vi "SA40144D.20210528 Devices + BG.vi"() -> ()   [LabVIEW 2020]
uses:
  <vilib>/Analysis/baseanly.llb/Mean (DBL).vi
  <userlib>/_OpenG.lib/file/file.llb/Build Path - Traditional__ogtk.vi
  <userlib>/LevyLab/LV to ITX/Data/Data.lvclass
  <userlib>/LevyLab/XY Utilities/xy_utilities.lvlib
  <vilib>/Analysis/NI_AALBase.lvlib
panel:
  out "G2T BG vs t":T1(graph)
  in  "Temps to keep (Lifespan)":i32=26
  out "Lifespan vs Temp (hrs)":cluster{i32[], dbl[]}[](graph)
  out "E_a":dbl[](array[numeric])
  out "Arrhenius":T1(graph)
  in  "Temps to keep (Arrhenius fit)":i32=26
  out "G2T vs t":T1(graph)
  out "G4T vs t":T1(graph)
  out "G2T vs t 2D":T1(graph)
  out "G4T vs t  2D":T1(graph)
  out "Temp vs t":T1(graph)
  in  "Source Voltage":dbl=0.1
  in  "Init Temp":i32=275
  in  "Temp Step":i32=5
  in  "Final Temp":i32=400
  in  "Data File":path=path "G:/My Drive/ansom/Data/PPMS 2/SA40144D.20210601/00 - Air Test/SA40144D.20210601.275K.dat"
  in  "Trimming":i32=400
  in  "Update":bool
  in  "OK":bool
  out "error out":errorcluster
  in  "error in (no error)":errorcluster
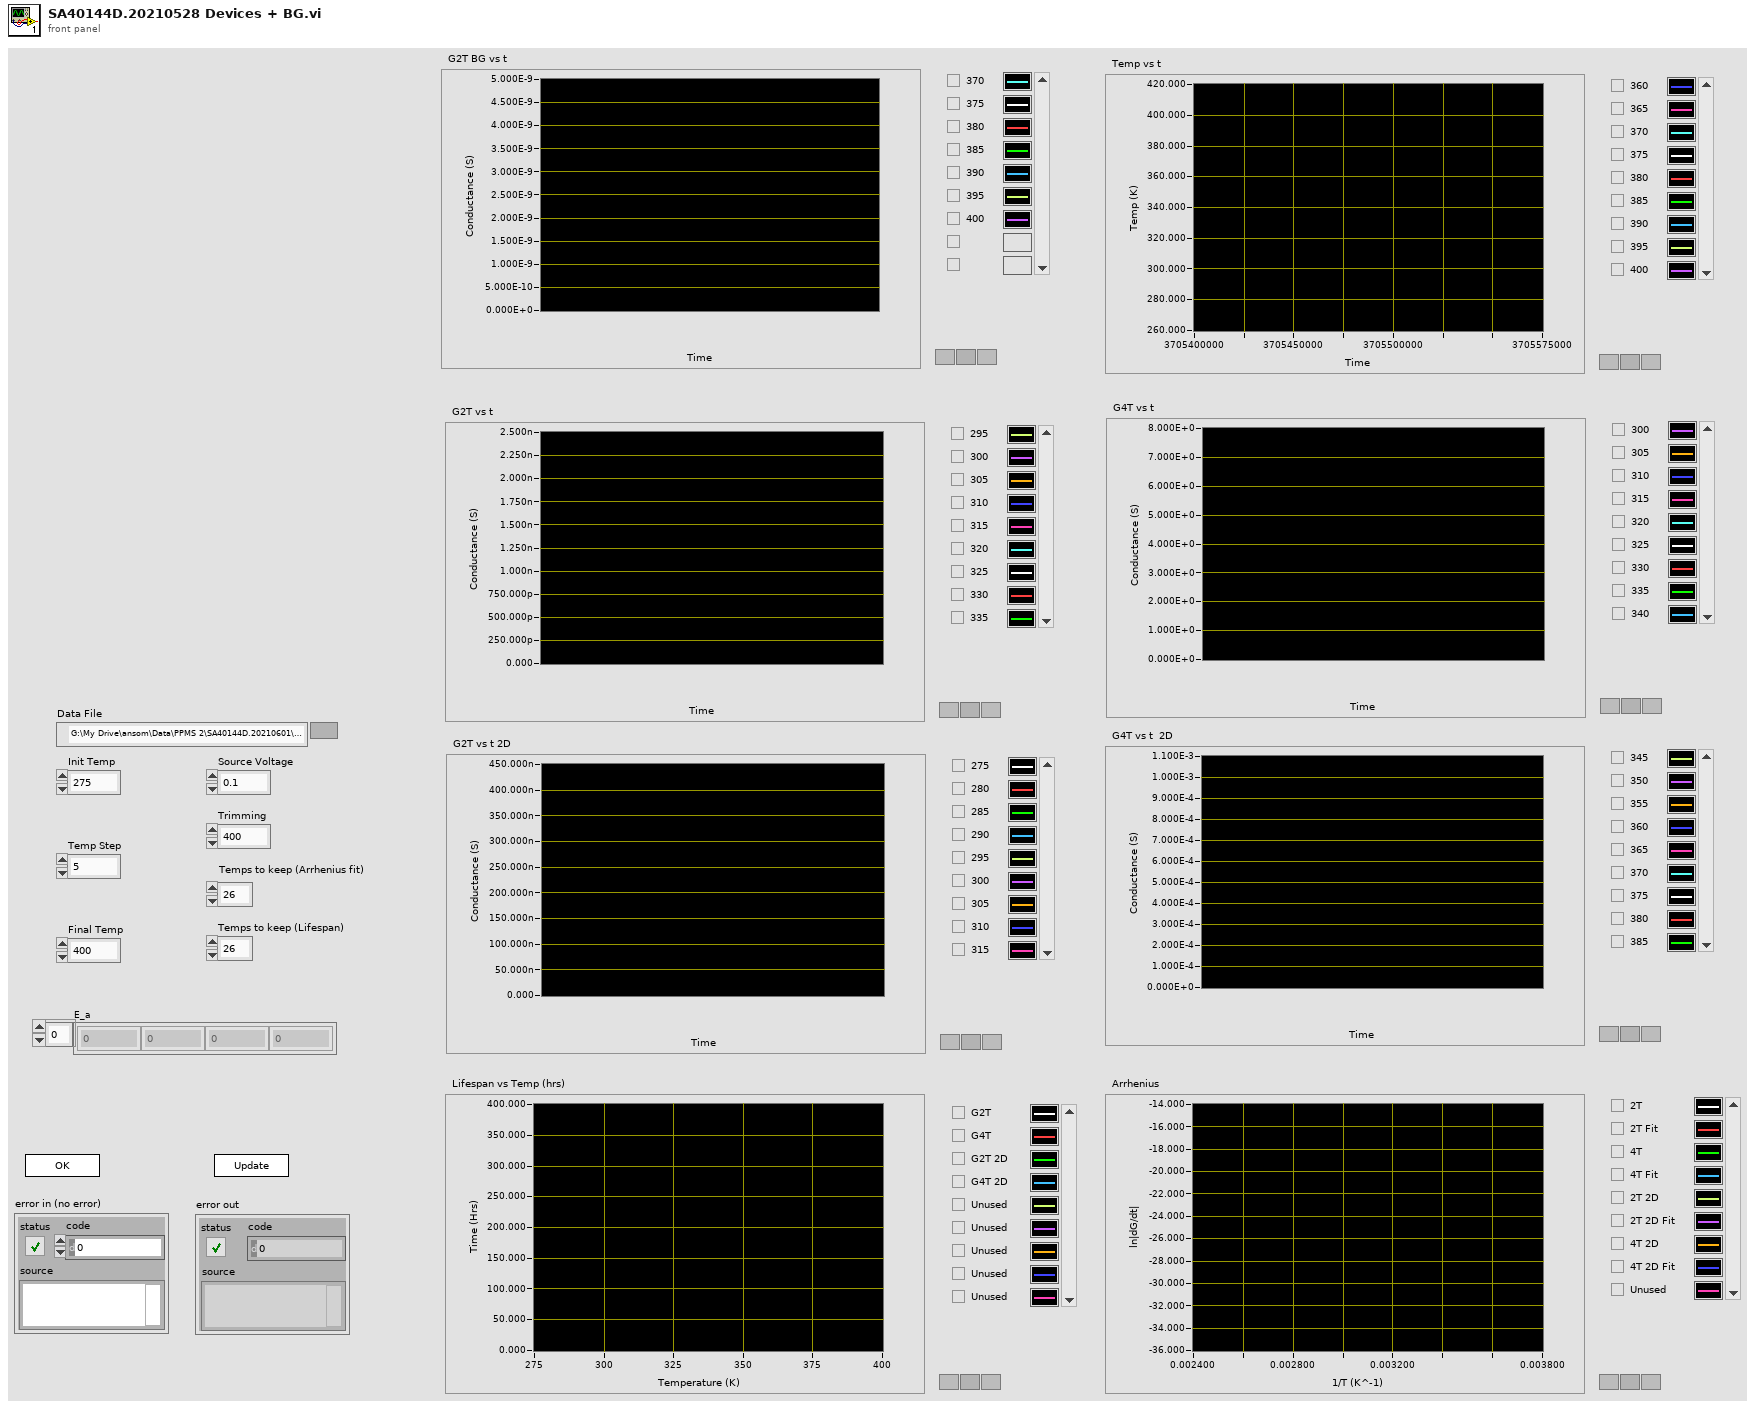
[diagram p1: front panel]
types:
  T1 = cluster{"Data":dbl[], "Best Exponential Fit":dbl[]}[]
  T2 = enum32{"Invalid", "Standard", "Closed", "Hidden", "Minimized", "Maximized"}
  T3 = enum32{"invalid app kind", "Development System", "Run Time System", "Student Edition", "Embedded LabVIEW", "Evaluation", "Custom"}
  T4 = cluster{"Core":cluster{"Current VI Reference":refnum<vi>, "Close Panel on Exit?":bool}, "G2T 1D":cluster{dbl[], dbl[]}[], "G4T 1D":cluster{dbl[], dbl[]}[], "G2T 2D":cluster{dbl[], dbl[]}[], "G4T 2D":cluster{dbl[], dbl[]}[], "Temp":cluster{dbl[], dbl[]}[], "G2T BG":cluster{dbl[], dbl[]}[], "Source Voltage":dbl, "Final Temp":i32, "Init Temp":i32, "Temp Step":i32, "Data File":path, "Trimming":i32}
  T5 = cluster{"Current VI Reference":refnum<vi>, "Close Panel on Exit?":bool}
  T6 = typedef "Data.lvclass/Dictionary--cluster.ctl" = cluster{"key":string, "value":variant}
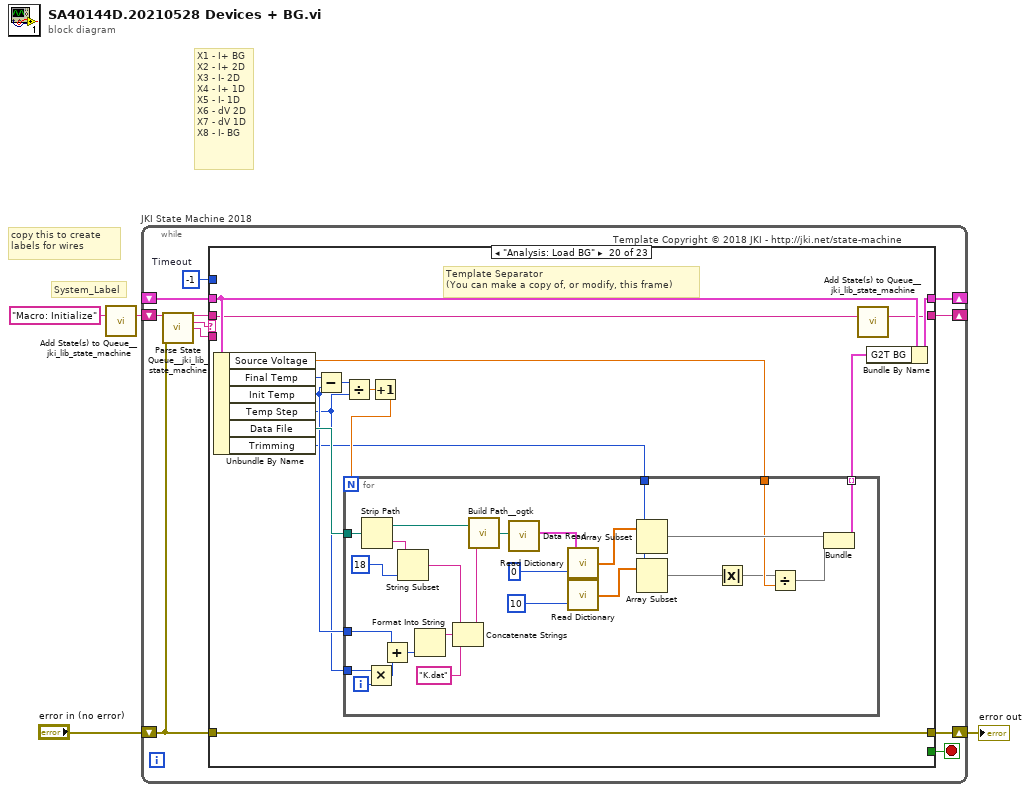
[diagram p0: block diagram]
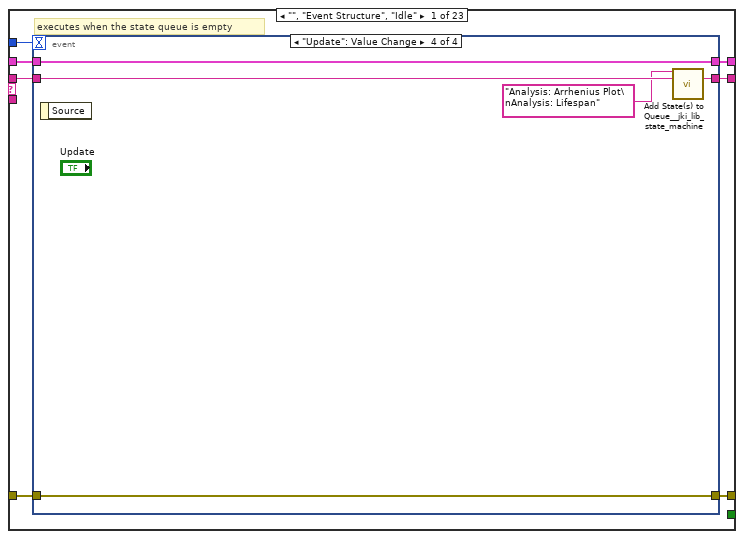
[diagram p2: hidden frame]
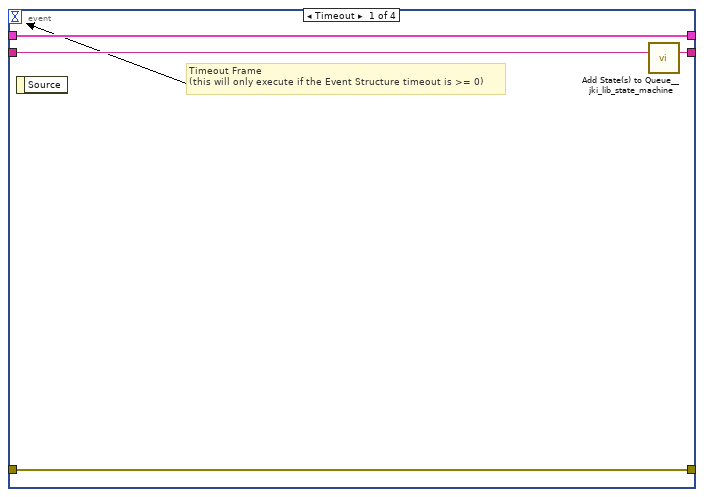
[diagram p3: hidden frame]
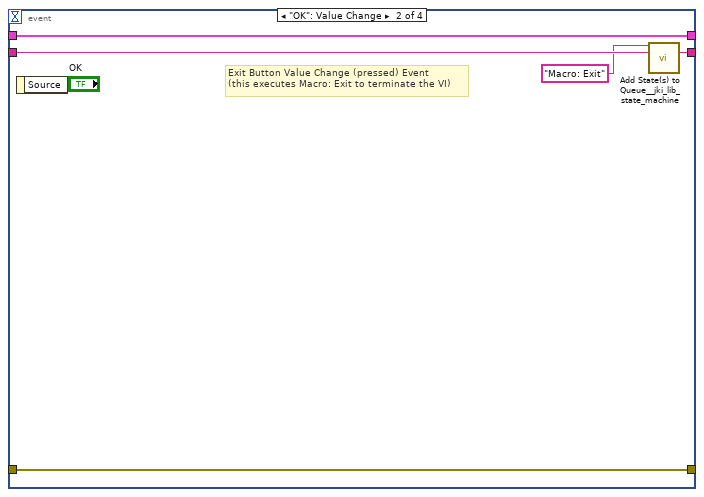
[diagram p4: hidden frame]
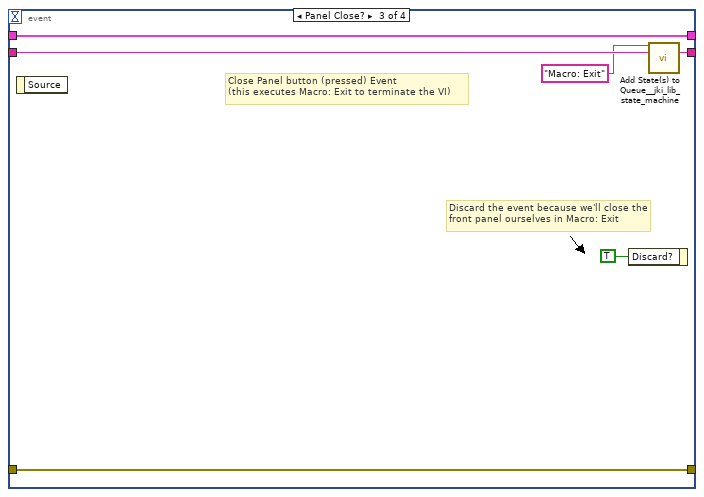
[diagram p5: hidden frame]
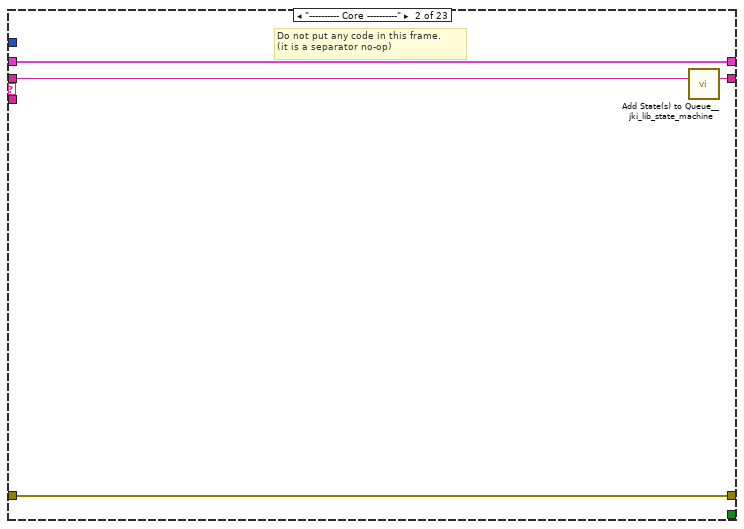
[diagram p6: hidden frame]
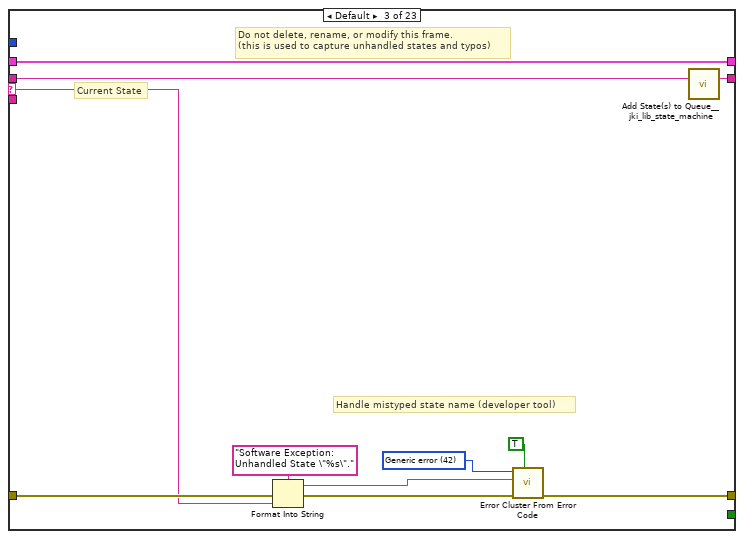
[diagram p7: hidden frame]
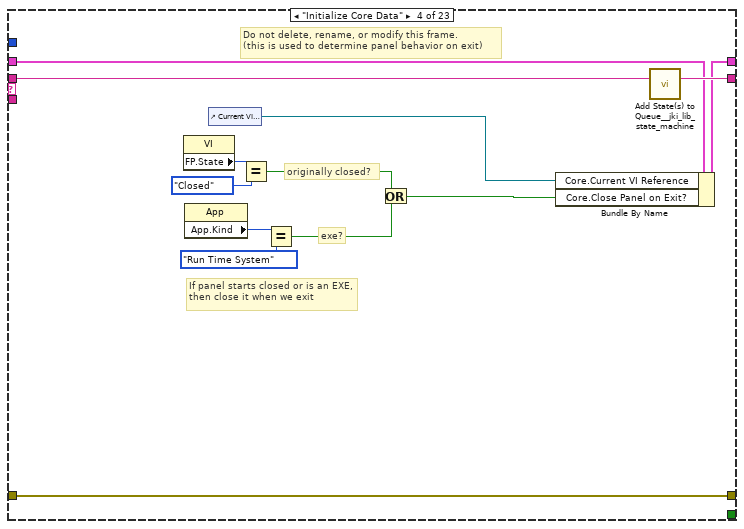
[diagram p8: hidden frame]
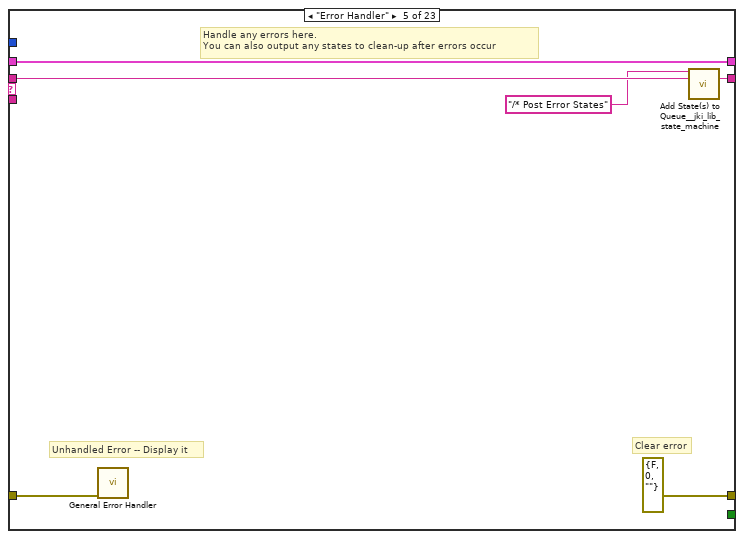
[diagram p9: hidden frame]
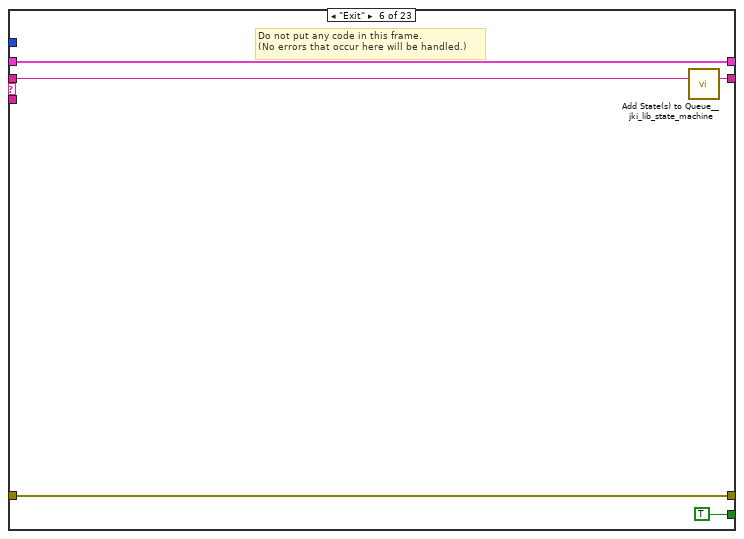
[diagram p10: hidden frame]
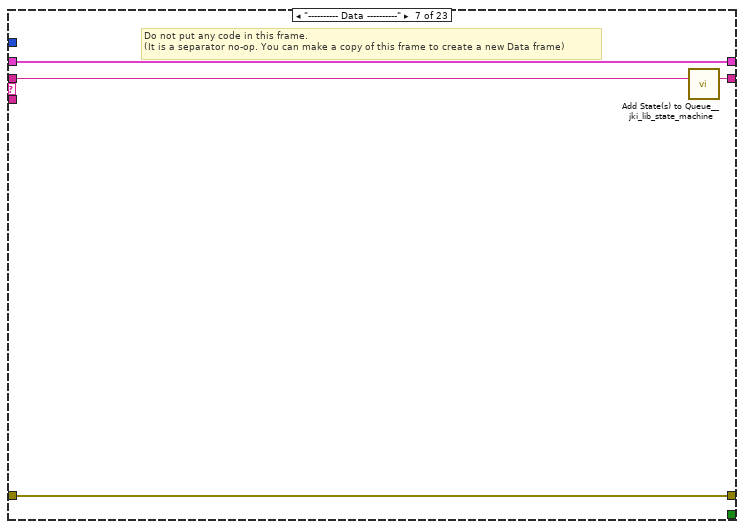
[diagram p11: hidden frame]
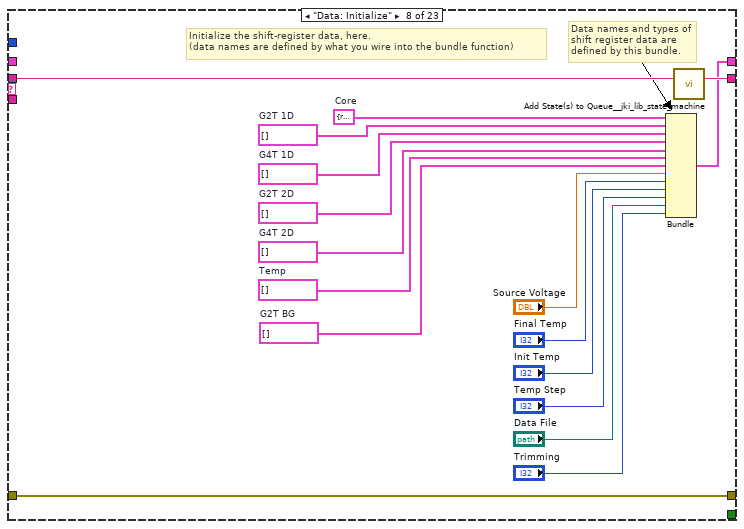
[diagram p12: hidden frame]
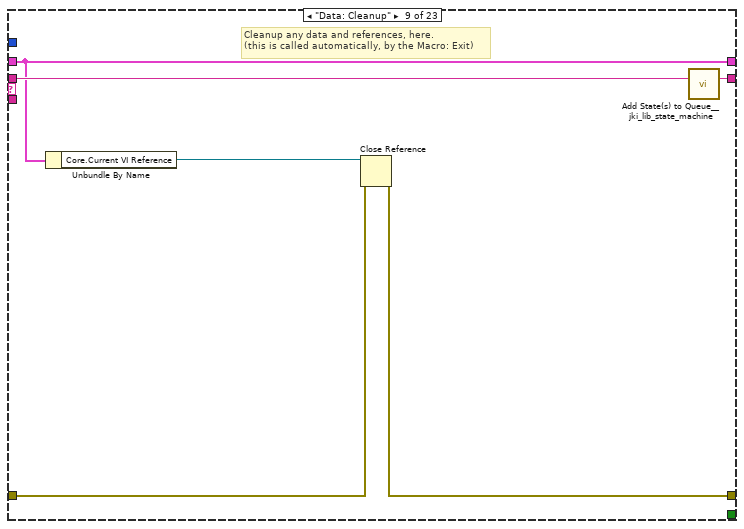
[diagram p13: hidden frame]
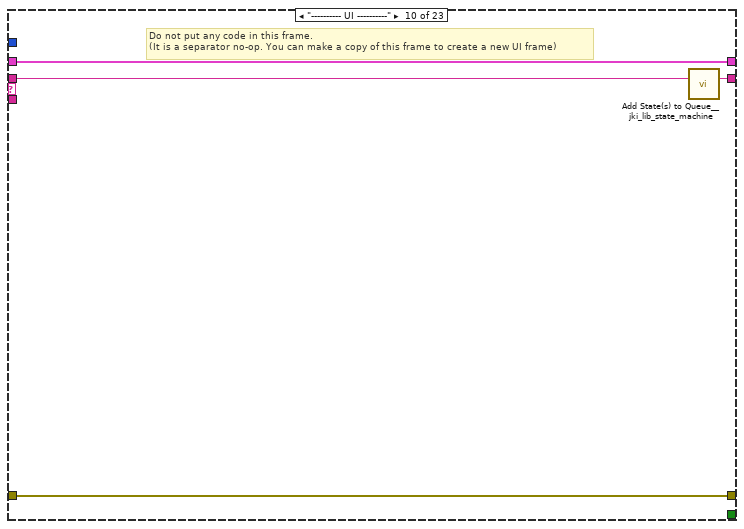
[diagram p14: hidden frame]
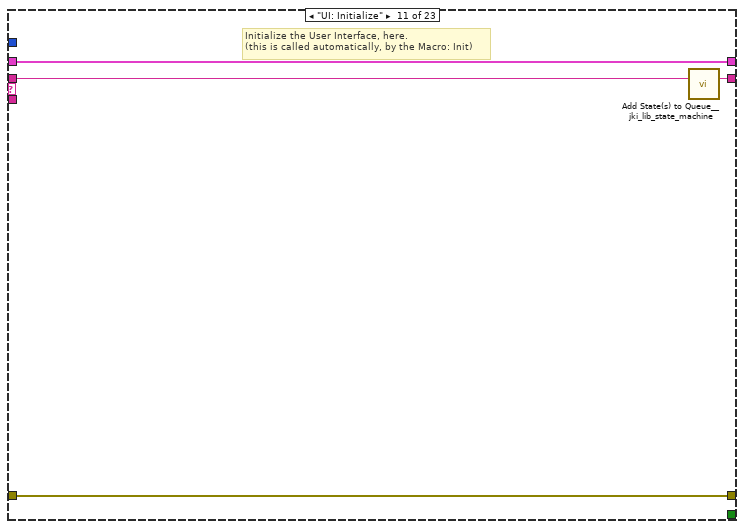
[diagram p15: hidden frame]
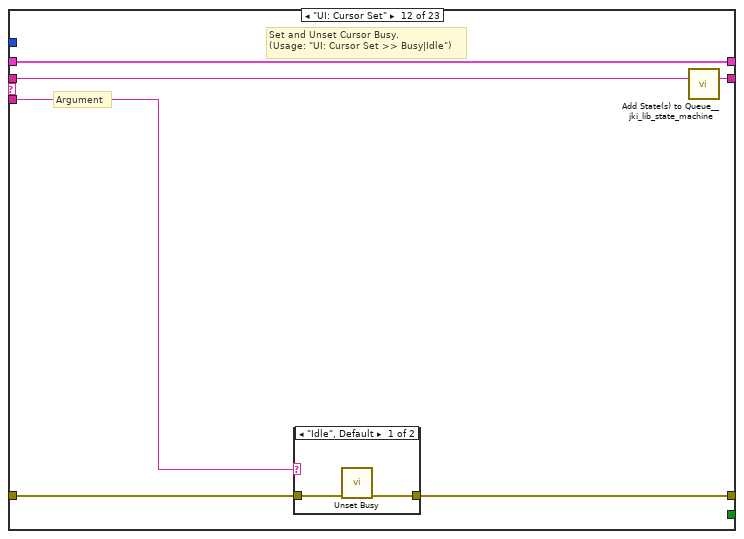
[diagram p16: hidden frame]
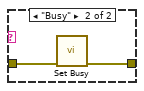
[diagram p17: hidden frame]
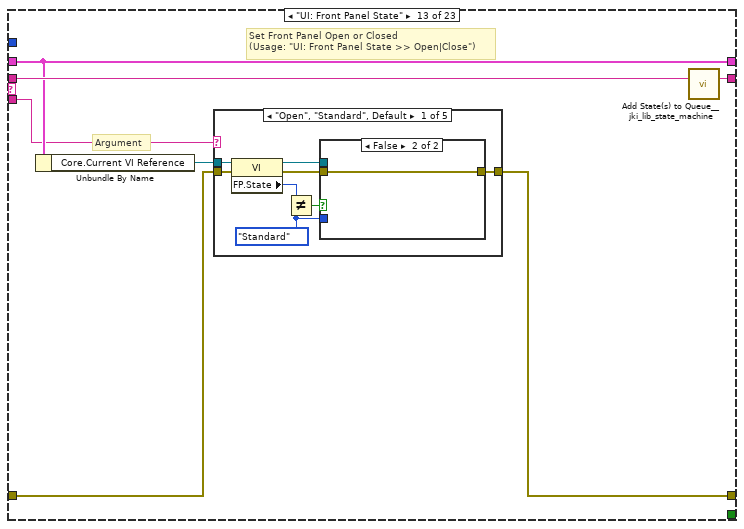
[diagram p18: hidden frame]
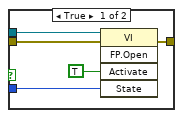
[diagram p19: hidden frame]
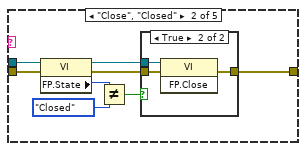
[diagram p20: hidden frame]
diagram:
  # "X1 - I+ BG\nX2 - I+ 2D\nX3 - I- 2D\nX4 - I+ 1D\nX5 - I- 1D\nX6 - dV 2D\nX7 - dV 1D\nX8 - I- BG"
  # "copy this to create labels for wires"
  # "System_Label"
  n1 = call <vilib>:"Add State(s) to Queue__jki_lib_state_machine.vi"("State(s) in (\"\")"="Macro: Initialize") -> ("States Out"=w4:string)  [unwired: 14 in]
  n2 = while "JKI State Machine 2018" {
    shift-right: [w8] -> _
    shift-left: _ -> [w7]
    shift-right: [w11] -> w1
    shift-left: "error in (no error)" -> [w5]
    shift-right: [w10] -> _
    shift-left: w4 -> [w12]
    stop <- w9 stop-if-true
    w6 = -1  # Timeout
    # "Template Copyright © 2018 JKI - http://jki.net/state-machine"
    n3 = call <vilib>:"Parse State Queue__jki_lib_state_machine.vi"("State Queue"=w12, "Error In (no error)"=w5) -> ("Remaining States"=w14:string, "Current State"=w15:string, "Arguments"=w13:string)  [unwired: 11 in]
    n4 = case shown="\"Analysis: Load BG\"" w15 {
      selector: w15 -> [_ _ w47 _ _ _ _ _ _ _ _ _ _ _ _ _ _ _ _ _ _ _ _]
      tunnel: w14 -> [w22 w46 w51 w70 w76 w81 w85 w102 w108 w112 w116 w122 w133 w202 w207 w217 w221 w238 w290 w323 w373 w417 w474]
      tunnel: w13 -> [_ _ _ _ _ _ _ _ _ _ _ w117 w127 _ _ _ _ _ _ _ _ _ _]
      tunnel: w7 -> [w20 w43 w49 w63 w73 w79 w82 _ w103 w109 w114 w120 w129 w199 w204 w214 w218 w232 w275 w325 w370 w414 w454]
      tunnel: [w19 w44 w53 w67 errorcluster {"status"=FALSE, "code"=0, "source"=""} ("error out") w78 w83 w99 w104 w110 w113 w118 w130 w200 w205 w215 w219 w234 w288 w337 w371 w415 w472] -> w11
      tunnel: w5 -> [w18 w44 w52 w67 w72 w78 w83 w99 w105 w110 w113 w119 w131 w200 w205 w215 w219 w234 w288 w337 w371 w415 w472]
      tunnel: [w21 w45 w50 w69 w75 w80 w84 w101 w107 w111 w115 w121 w132 w201 w206 w216 w220 w237 w289 w324 w372 w416 w473] -> w10
      tunnel: [_ _ _ _ _ TRUE _ _ _ _ _ _ _ _ _ _ _ _ _ _ _ _ _] -> w9
      tunnel: [w17 w43 w49 w68 w73 w79 w82 w100 w103 w109 w114 w120 w129 w199 w204 w214 w218 w233 w276 w326 w370 w414 w454] -> w8
      tunnel: w6 -> [w16 _ _ _ _ _ _ _ _ _ _ _ _ _ _ _ _ _ _ _ _ _ _]
      frame "", "Event Structure", "Idle" {
        # "executes when the state queue is empty"
        n5 = event shown="[3] \"Update\": Value Change" {
          selector: _ -> [_ _ _ _]
          dyn-events: _ -> [_ _ _ _]
          timeout: w16 -> [_ _ _ _]
          tunnel: w22 -> [w26 w31 w37 w41]
          tunnel: [w25 w30 w36 w40] -> w21
          tunnel: w20 -> [w23 w28 w34 w42]
          tunnel: [w24 w29 w35 w38] -> w19
          tunnel: w18 -> [w24 w29 w35 w38]
          tunnel: [w23 w28 w34 w42] -> w17
          event Timeout {
            # "Timeout Frame\n(this will only execute if the Event Structure timeout is >= 0)"
            n6 = event-data() -> ()  [unwired: 1 in, 1 out]
            n7 = call <vilib>:"Add State(s) to Queue__jki_lib_state_machine.vi"("State(s) in (\"\")"=w26) -> ("States Out"=w25:string)  [unwired: 14 in]
          }
          event "OK": Value Change {
            # "Exit Button Value Change (pressed) Event\n(this executes Macro: Exit to terminate the VI)"
            n8 = event-data() -> ()  [unwired: 1 in, 1 out]
            n9 = call <vilib>:"Add State(s) to Queue__jki_lib_state_machine.vi"("State(s) in Front (\"\")"="Macro: Exit", "State(s) in (\"\")"=w31) -> ("States Out"=w30:string)  [unwired: 13 in]
          }
          event Panel Close? {
            # "Discard the event because we'll close the front panel ourselves in Macro: Exit"
            # "Close Panel button (pressed) Event\n(this executes Macro: Exit to terminate the VI)"
            n10 = event-data() -> ()  [unwired: 1 in, 1 out]
            n11 = event-data("Discard?"=TRUE) -> ()  [unwired: 1 in, 1 out]
            n12 = call <vilib>:"Add State(s) to Queue__jki_lib_state_machine.vi"("State(s) in Front (\"\")"="Macro: Exit", "State(s) in (\"\")"=w37) -> ("States Out"=w36:string)  [unwired: 13 in]
          }
          event "Update": Value Change {
            n13 = event-data() -> ()  [unwired: 1 in, 1 out]
            n14 = call <vilib>:"Add State(s) to Queue__jki_lib_state_machine.vi"("State(s) in Front (\"\")"="Analysis: Arrhenius Plot\nAnalysis: Lifespan" ("State(s) in Front (\"\")"), "State(s) in (\"\")"=w41) -> ("States Out"=w40:string)  [unwired: 13 in]
          }
        }
      }
      frame "---------- Core ----------" {
        # "Do not put any code in this frame.\n(it is a separator no-op)"
        n15 = call <vilib>:"Add State(s) to Queue__jki_lib_state_machine.vi"("State(s) in (\"\")"=w46) -> ("States Out"=w45:string)  [unwired: 14 in]
      }
      frame Default {
        w56 = 42 items=["No error", "Argument error", "Memory is full", "Out of zone", "End of file", "File already open", "Generic file I/O error", "File not found", "File permission error", "Disk is full", "Duplicate path", "Too many files open", "System feature not enabled", "Resource file not found", "Cannot add resource", "Resource not found", "Image not found", "Image memory error", "Pen does not exist", "Config type invalid", "Config token not found", "Config parse error", "Config memory error", "Bad external code format", "Bad external code offset", "External code not present", "Null window", "Destroy window error", "Null menu", "Print aborted", "Bad print record", "Print driver error", "Windows error during printing", "Memory error during printing", "Print dialog error", "Generic print error", "Invalid device refnum", "Device not found", "Device parameter error", "Device unit error", "Cannot open device", "Device call aborted", "Generic error", "Cancelled by user", "Object ID too low", "Object ID too high", "Object not in heap", "Unknown heap", "Unknown object (invalid DefProc)", "Unknown object (DefProc not in table)", "Message out of range", "Invalid (null) method", "Unknown message", "Manager call not supported", "Bad address", "Network operation in progress", "Network operation timed out", "Connection is busy", "Network attribute not supported", "Network error", "Address in use", "System out of memory", "Connection aborted", "Connection refused", "Not connected", "Already connected", "Connection closed", "Initialization error (interapplication manager)", "Bad occurrence", "Wait on unbound occurrence handler", "Occurrence queue overflow", "Datalog type conflict", "Unused", "Unrecognized type (interapplication manager)", "Memory corrupt", "Failed to make temporary DLL", "Old CIN version", "Drag socket not found", "Failed to load drop-object", "Failed to register OLE object", "Failed to release OLE object", "Format specifier type mismatch", "Unknown format specifier", "Too few format specifiers", "Too many format specifiers", "Scan failed", "Newer CIN version", "Error converting to variant", "Runtime menu error", "Password tampered", "Variant attribute not found", "Incompatible variant data type", "Event data is not available", "Event Store is not present", "Occurrence is not found", "Event Queue is not created", "Event info is not available", "Refnum passed is NULL", "Error retrieving Class GUID", "Error retrieving CoClass GUID", "Error retrieving TypeLib GUID.", "Bad built application magic bytes.", "Specific driver is different from the specific driver associated with the Logical Name.", "There is no session opened to the class driver.", "Max Error", "MAX - Error with config objects", "MAX - Error loading configuration", "MAX - Group not supported"]
        # "Current State"
        # "Do not delete, rename, or modify this frame.\n(this is used to capture unhandled states and typos)"
        # "Handle mistyped state name (developer tool)"
        n16 = Format Into String(format string="Software Exception: Unhandled State \"%s\"." ("message"), error in=w52, w47) -> (resulting string=w55:string, error out=w54:errorcluster)  [unwired: 1 in]
        n17 = call <vilib>:"Error Cluster From Error Code.vi"("show call chain? (False)"=TRUE, "error in (no error)"=w54, "error message (\"\")"=w55, "error code (0)"=w56) -> ("error out"=w53:errorcluster)  [unwired: 5 in]
        n18 = call <vilib>:"Add State(s) to Queue__jki_lib_state_machine.vi"("State(s) in (\"\")"=w51) -> ("States Out"=w50:string)  [unwired: 14 in]
      }
      frame "Initialize Core Data" {
        # "Do not delete, rename, or modify this frame.\n(this is used to determine panel behavior on exit)"
        # "originally closed?"
        # "exe?"
        # "If panel starts closed or is an EXE, then close it when we exit"
        n19 = property class="VI"() -> ("FP.State"=w60:T2)  [unwired: 2 in, 2 out]
        n20 = property class="App"() -> ("App.Kind"=w66:T3)  [unwired: 2 in, 2 out]
        n21 = control-ref of="Current VI Reference"() -> (w61:refnum<vi>)
        n22 = Equal?(x=w60, y=T2."Closed" ("Front Panel Window:State")) -> (x = y?=w58:bool)
        n23 = Equal?(x=w66, y=T3."Run Time System" ("Application:Kind")) -> (x = y?=w64:bool)
        n24 = Or(x=w58, y=w64) -> (x .or. y?=w62:bool)
        n25 = Bundle By Name(cluster=w63, "Core.Current VI Reference"=w61, "Core.Close Panel on Exit?"=w62) -> (w68:T4)
        n26 = call <vilib>:"Add State(s) to Queue__jki_lib_state_machine.vi"("State(s) in (\"\")"=w70) -> ("States Out"=w69:string)  [unwired: 14 in]
      }
      frame "Error Handler" {
        # "Unhandled Error -- Display it"
        # "Handle any errors here.\nYou can also output any states to clean-up after errors occur"
        # "Clear error"
        n27 = call <vilib>:"General Error Handler.vi"("error in (no error)"=w72) -> ()  [unwired: 10 in, 5 out]
        n28 = call <vilib>:"Add State(s) to Queue__jki_lib_state_machine.vi"("State(s) in Front (\"\")"="/* Post Error States", "State(s) in (\"\")"=w76) -> ("States Out"=w75:string)  [unwired: 13 in]
      }
      frame "Exit" {
        # "Do not put any code in this frame.\n(No errors that occur here will be handled.)"
        n29 = call <vilib>:"Add State(s) to Queue__jki_lib_state_machine.vi"("State(s) in (\"\")"=w81) -> ("States Out"=w80:string)  [unwired: 14 in]
      }
      frame "---------- Data ----------" {
        # "Do not put any code in this frame.\n(It is a separator no-op. You can make a copy of this frame to create a new Data frame)"
        n30 = call <vilib>:"Add State(s) to Queue__jki_lib_state_machine.vi"("State(s) in (\"\")"=w85) -> ("States Out"=w84:string)  [unwired: 14 in]
      }
      frame "Data: Initialize" {
        w86 = cluster{dbl[], dbl[]}[] []  # G2T BG
        w87 = cluster{dbl[], dbl[]}[] []  # Temp
        w96 = cluster{dbl[], dbl[]}[] []  # G4T 2D
        w95 = cluster{dbl[], dbl[]}[] []  # G2T 2D
        w94 = cluster{dbl[], dbl[]}[] []  # G4T 1D
        w93 = cluster{dbl[], dbl[]}[] []  # G2T 1D
        w98 = T5 {"Current VI Reference"=refnum, "Close Panel on Exit?"=FALSE}  # Core
        # "Data names and types of shift register data are defined by this bundle."
        # "Initialize the shift-register data, here.\n(data names are defined by what you wire into the bundle function)"
        n31 = Bundle("Core"=w98, "G2T 1D"=w93, "G4T 1D"=w94, "G2T 2D"=w95, "G4T 2D"=w96, "Temp"=w87, "G2T BG"=w86, "Source Voltage"="Source Voltage", "Final Temp"="Final Temp", "Init Temp"="Init Temp", "Temp Step"="Temp Step", "Data File"="Data File", "Trimming"="Trimming") -> (w100:T4)  [unwired: 1 in]
        n32 = call <vilib>:"Add State(s) to Queue__jki_lib_state_machine.vi"("State(s) in (\"\")"=w102) -> ("States Out"=w101:string)  [unwired: 14 in]
      }
      frame "Data: Cleanup" {
        # "Cleanup any data and references, here.\n(this is called automatically, by the Macro: Exit)"
        n33 = Unbundle By Name(w103) -> ("Core.Current VI Reference"=w106:refnum<vi>)
        n34 = Close Reference(reference=w106, error in (no error)=w105) -> (error out=w104:errorcluster)
        n35 = call <vilib>:"Add State(s) to Queue__jki_lib_state_machine.vi"("State(s) in (\"\")"=w108) -> ("States Out"=w107:string)  [unwired: 14 in]
      }
      frame "---------- UI ----------" {
        # "Do not put any code in this frame.\n(It is a separator no-op. You can make a copy of this frame to create a new UI frame)"
        n36 = call <vilib>:"Add State(s) to Queue__jki_lib_state_machine.vi"("State(s) in (\"\")"=w112) -> ("States Out"=w111:string)  [unwired: 14 in]
      }
      frame "UI: Initialize" {
        # "Initialize the User Interface, here.\n(this is called automatically, by the Macro: Init)"
        n37 = call <vilib>:"Add State(s) to Queue__jki_lib_state_machine.vi"("State(s) in (\"\")"=w116) -> ("States Out"=w115:string)  [unwired: 14 in]
      }
      frame "UI: Cursor Set" {
        # "Argument"
        # "Set and Unset Cursor Busy.\n(Usage: \"UI: Cursor Set >> Busy|Idle\")"
        n38 = case shown="\"Idle\", Default" w117 {
          tunnel: w119 -> [w124 w126]
          tunnel: [w123 w125] -> w118
          frame "Idle", Default {
            n39 = call <vilib>:"Unset Busy.vi"("error in (no error)"=w124) -> ("error out"=w123:errorcluster)  [unwired: 10 in]
          }
          frame "Busy" {
            n40 = call <vilib>:"Set Busy.vi"("error in (no error)"=w126) -> ("error out"=w125:errorcluster)  [unwired: 9 in, 1 out]
          }
        }
        n41 = call <vilib>:"Add State(s) to Queue__jki_lib_state_machine.vi"("State(s) in (\"\")"=w122) -> ("States Out"=w121:string)  [unwired: 14 in]
      }
      frame "UI: Front Panel State" {
        # "Argument"
        # "Set Front Panel Open or Closed\n(Usage: \"UI: Front Panel State >> Open|Close\")"
        n42 = Unbundle By Name(w129) -> ("Core.Current VI Reference"=w128:refnum<vi>)
        n43 = case shown="\"Open\", \"Standard\", Default" w127 {
          tunnel: w131 -> [w139 w154 w165 w178 w191]
          tunnel: [w141 w155 w167 w180 w193] -> w130
          tunnel: w128 -> [w140 w152 w166 w179 w192]
          frame "Open", "Standard", Default {
            w134 = T2."Standard" ("State")
            n44 = property class="VI"(reference=w140, error in=w139) -> (reference out=w137:refnum<vi>, error out=w138:errorcluster, "FP.State"=w136:T2)
            n45 = Not Equal?(x=w136, y=w134) -> (x != y?=w135:bool)
            n46 = case shown="False" w135 {
              tunnel: [w145 w147] -> w141
              tunnel: w138 -> [w144 w147]
              tunnel: w137 -> [w143 _]
              tunnel: w134 -> [w142 _]
              frame True {
                n47 = invoke class="VI" method="FP.Open"(reference=w143, error in=w144, "Activate"=TRUE, "State"=w142) -> (error out=w145:errorcluster)  [unwired: 1 in, 4 out]
              }
              frame False {
              }
            }
          }
          frame "Close", "Closed" {
            n48 = property class="VI"(reference=w152, error in=w154) -> (reference out=w151:refnum<vi>, error out=w153:errorcluster, "FP.State"=w149:T2)
            n49 = Not Equal?(x=w149, y=T2."Closed" ("Front Panel Window:State")) -> (x != y?=w148:bool)
            n50 = case shown="True" w148 {
              tunnel: [w156 w159] -> w155
              tunnel: w153 -> [w156 w158]
              tunnel: w151 -> [_ w157]
              frame False {
              }
              frame True {
                n51 = invoke class="VI" method="FP.Close"(reference=w157, error in=w158) -> (error out=w159:errorcluster)  [unwired: 1 in, 2 out]
              }
            }
          }
          frame "Hidden", "Hide" {
            w160 = T2."Hidden" ("State")
            n52 = property class="VI"(reference=w166, error in=w165) -> (reference out=w163:refnum<vi>, error out=w164:errorcluster, "FP.State"=w162:T2)
            n53 = Not Equal?(x=w162, y=w160) -> (x != y?=w161:bool)
            n54 = case shown="True" w161 {
              tunnel: [w171 w172] -> w167
              tunnel: w164 -> [w170 w172]
              tunnel: w163 -> [w169 _]
              tunnel: w160 -> [w168 _]
              frame True {
                n55 = invoke class="VI" method="FP.Open"(reference=w169, error in=w170, "State"=w168) -> (error out=w171:errorcluster)  [unwired: 2 in, 4 out]
              }
              frame False {
              }
            }
          }
          frame "Minimize", "Minimized" {
            w173 = T2."Minimized" ("State")
            n56 = property class="VI"(reference=w179, error in=w178) -> (reference out=w176:refnum<vi>, error out=w177:errorcluster, "FP.State"=w175:T2)
            n57 = Not Equal?(x=w175, y=w173) -> (x != y?=w174:bool)
            n58 = case shown="True" w174 {
              tunnel: [w184 w185] -> w180
              tunnel: w177 -> [w183 w185]
              tunnel: w176 -> [w182 _]
              tunnel: w173 -> [w181 _]
              frame True {
                n59 = invoke class="VI" method="FP.Open"(reference=w182, error in=w183, "State"=w181) -> (error out=w184:errorcluster)  [unwired: 2 in, 4 out]
              }
              frame False {
              }
            }
          }
          frame "Maximize", "Maximized" {
            w186 = T2."Maximized" ("State")
            n60 = property class="VI"(reference=w192, error in=w191) -> (reference out=w189:refnum<vi>, error out=w190:errorcluster, "FP.State"=w188:T2)
            n61 = Not Equal?(x=w188, y=w186) -> (x != y?=w187:bool)
            n62 = case shown="True" w187 {
              tunnel: [w197 w198] -> w193
              tunnel: w190 -> [w196 w198]
              tunnel: w189 -> [w195 _]
              tunnel: w186 -> [w194 _]
              frame True {
                n63 = invoke class="VI" method="FP.Open"(reference=w195, error in=w196, "State"=w194) -> (error out=w197:errorcluster)  [unwired: 2 in, 4 out]
              }
              frame False {
              }
            }
          }
        }
        n64 = call <vilib>:"Add State(s) to Queue__jki_lib_state_machine.vi"("State(s) in (\"\")"=w133) -> ("States Out"=w132:string)  [unwired: 14 in]
      }
      frame "---------- Macro ----------" {
        # "Do not put any code in this frame.\n(It is a separator no-op. You can make a copy of this frame to create a new Macro frame)"
        n65 = call <vilib>:"Add State(s) to Queue__jki_lib_state_machine.vi"("State(s) in (\"\")"=w202) -> ("States Out"=w201:string)  [unwired: 14 in]
      }
      frame "Macro: Initialize" {
        # "Initialization Macro\n(This is called once, when the VI starts)"
        n66 = call <vilib>:"Add State(s) to Queue__jki_lib_state_machine.vi"("State(s) in Front (\"\")"="Data: Initialize\nInitialize Core Data\nUI: Initialize\nUI: Front Panel State >> Open\nAnalysis: Load 1D\nAnalysis: Load 2D\nAnalysis: Load BG\nAnalysis: Plot G vs t\nAnalysis: Arrhenius Plot\nAnalysis: Lifespan", "State(s) in (\"\")"=w207) -> ("States Out"=w206:string)  [unwired: 13 in]
      }
      frame "Macro: Exit" {
        # "Exit Macro\n(This is called once, when the VI exits)"
        n67 = Unbundle By Name(w214) -> ("Core.Close Panel on Exit?"=w213:bool)
        n68 = Select(t="UI: Front Panel State >> Close", s=w213, f="") -> (s? t:f=w210:string)
        n69 = call <vilib>:"Add State(s) to Queue__jki_lib_state_machine.vi"("State(s) in (\"\")"=w210, "State(s) at Back (\"\")"="Data: Cleanup\nExit") -> ("States Out"=w208:string)  [unwired: 13 in]
        n70 = call <vilib>:"Add State(s) to Queue__jki_lib_state_machine.vi"("State(s) in Front (\"\")"=w208, "State(s) in (\"\")"=w217) -> ("States Out"=w216:string)  [unwired: 13 in]
      }
      frame "---------- Analysis ----------" {
        # "Template Separator\n(You can make a copy of, or modify, this frame)"
        n71 = call <vilib>:"Add State(s) to Queue__jki_lib_state_machine.vi"("State(s) in (\"\")"=w221) -> ("States Out"=w220:string)  [unwired: 14 in]
      }
      frame "Analysis: Load 1D" {
        n72 = Unbundle By Name(w232) -> ("Source Voltage"=w231:dbl, "Final Temp"=w228:i32, "Init Temp"=w225:i32, "Temp Step"=w224:i32, "Data File"=w226:path, "Trimming"=w223:i32)
        n73 = Subtract(x=w228, y=w225) -> (x-y=w235:i32)
        n74 = Divide(x=w235, y=w224) -> (x/y=w236:dbl)
        n75 = Increment(x=w236) -> (x+1=w227:dbl)
        n76 = for {
          N: w227 -> [_]
          tunnel: w231 -> [w244]
          tunnel: [w262] -> w230 mode=indexing
          tunnel: [w261] -> w229 mode=indexing
          tunnel: w226 -> [w260]
          tunnel: w225 -> [w259]
          tunnel: w224 -> [w258]
          tunnel: w223 -> [w257]
          tunnel: [w254] -> w222 mode=indexing
          i -> [w265]
          n77 = Strip Path(path=w260) -> (stripped path=w270:path, name=w269:string)
          n78 = Multiply(x=w258, y=w265) -> (x*y=w266:i32)
          n79 = Add(x=w259, y=w266) -> (x+y=w271:i32)
          n80 = String Subset(string=w269, length (rest)=18) -> (substring=w267:string)  [unwired: 1 in]
          n81 = Format Into String(w271) -> (resulting string=w273:string)  [unwired: 3 in, 1 out]
          n82 = Concatenate Strings(w267, w273, "K.dat" ("string")) -> (w272:string)
          n83 = call-poly <userlib>:"Build Path__ogtk.vi"("name or relative path"=w272, "base path"=w270) -> ("appended path"=w274:path)
          n84 = call <userlib>:"Data Read.vi"("path"=w274) -> ("Data (Dictionary)"=w253:T6[])  [unwired: 7 in, 3 out]
          n85 = call "Read Dictionary.vi"("Numeric"=0, "Dictionary In"=w253) -> ("data"=w249:dbl[])
          n86 = call "Read Dictionary.vi"("Numeric"=7 ("index"), "Dictionary In"=w253) -> ("data"=w245:dbl[])
          n87 = call "Read Dictionary.vi"("Numeric"=9, "Dictionary In"=w253) -> ("data"=w248:dbl[])
          n88 = call "Read Dictionary.vi"("Numeric"=1, "Dictionary In"=w253) -> ("data"=w247:dbl[])
          n89 = Array Subset(array=w249, index=w257) -> (w256:dbl[])  [unwired: 1 in]
          n90 = Array Subset(array=w245, index=w257) -> (w243:dbl[])  [unwired: 1 in]
          n91 = Array Subset(array=w248, index=w257) -> (w242:dbl[])  [unwired: 1 in]
          n92 = Divide(x=w243, y=w244) -> (x/y=w264:dbl[])
          n93 = Absolute Value(x=w264) -> (abs(x)=w241:dbl[])
          n94 = Array Subset(array=w247) -> (w255:dbl[])  [unwired: 2 in]
          n95 = Divide(x=w243, y=w242) -> (x/y=w239:dbl[])
          n96 = Bundle(w256, w241) -> (w262:cluster{dbl[], dbl[]})  [unwired: 1 in]
          n97 = Bundle(w256, w255) -> (w254:cluster{dbl[], dbl[]})  [unwired: 1 in]
          n98 = Absolute Value(x=w239) -> (abs(x)=w240:dbl[])
          n99 = Bundle(w256, w240) -> (w261:cluster{dbl[], dbl[]})  [unwired: 1 in]
        }
        n100 = call <vilib>:"Add State(s) to Queue__jki_lib_state_machine.vi"("State(s) in (\"\")"=w238) -> ("States Out"=w237:string)  [unwired: 14 in]
        n101 = Bundle By Name(cluster=w232, "G2T 1D"=w230, "G4T 1D"=w229, "Temp"=w222) -> (w233:T4)
      }
      frame "Analysis: Load 2D" {
        n102 = Unbundle By Name(w275) -> ("Source Voltage"=w285:dbl, "Final Temp"=w282:i32, "Init Temp"=w279:i32, "Temp Step"=w278:i32, "Data File"=w280:path, "Trimming"=w277:i32)
        n103 = Subtract(x=w282, y=w279) -> (x-y=w286:i32)
        n104 = Divide(x=w286, y=w278) -> (x/y=w287:dbl)
        n105 = Increment(x=w287) -> (x+1=w281:dbl)
        n106 = for {
          N: w281 -> [_]
          tunnel: w285 -> [w294]
          tunnel: [w309] -> w284 mode=indexing
          tunnel: [w308] -> w283 mode=indexing
          tunnel: w280 -> [w307]
          tunnel: w279 -> [w306]
          tunnel: w278 -> [w305]
          tunnel: w277 -> [w304]
          i -> [w313]
          n107 = Strip Path(path=w307) -> (stripped path=w318:path, name=w317:string)
          n108 = Multiply(x=w305, y=w313) -> (x*y=w314:i32)
          n109 = Add(x=w306, y=w314) -> (x+y=w319:i32)
          n110 = String Subset(string=w317, length (rest)=18) -> (substring=w315:string)  [unwired: 1 in]
          n111 = Format Into String(w319) -> (resulting string=w321:string)  [unwired: 3 in, 1 out]
          n112 = Concatenate Strings(w315, w321, "K.dat" ("string")) -> (w320:string)
          n113 = call-poly <userlib>:"Build Path__ogtk.vi"("name or relative path"=w320, "base path"=w318) -> ("appended path"=w322:path)
          n114 = call <userlib>:"Data Read.vi"("path"=w322) -> ("Data (Dictionary)"=w302:T6[])  [unwired: 7 in, 3 out]
          n115 = call "Read Dictionary.vi"("Numeric"=0, "Dictionary In"=w302) -> ("data"=w301:dbl[])
          n116 = call "Read Dictionary.vi"("Numeric"=6 ("index"), "Dictionary In"=w302) -> ("data"=w299:dbl[])
          n117 = call "Read Dictionary.vi"("Numeric"=8, "Dictionary In"=w302) -> ("data"=w300:dbl[])
          n118 = Array Subset(array=w301, index=w304) -> (w303:dbl[])  [unwired: 1 in]
          n119 = Array Subset(array=w299, index=w304) -> (w295:dbl[])  [unwired: 1 in]
          n120 = Array Subset(array=w300, index=w304) -> (w293:dbl[])  [unwired: 1 in]
          n121 = Divide(x=w295, y=w294) -> (x/y=w311:dbl[])
          n122 = Absolute Value(x=w311) -> (abs(x)=w291:dbl[])
          n123 = Divide(x=w295, y=w293) -> (x/y=w312:dbl[])
          n124 = Bundle(w303, w291) -> (w309:cluster{dbl[], dbl[]})  [unwired: 1 in]
          n125 = Absolute Value(x=w312) -> (abs(x)=w292:dbl[])
          n126 = Bundle(w303, w292) -> (w308:cluster{dbl[], dbl[]})  [unwired: 1 in]
        }
        n127 = call <vilib>:"Add State(s) to Queue__jki_lib_state_machine.vi"("State(s) in (\"\")"=w290) -> ("States Out"=w289:string)  [unwired: 14 in]
        n128 = Bundle By Name(cluster=w275, "G2T 2D"=w284, "G4T 2D"=w283) -> (w276:T4)
      }
      frame "Analysis: Load BG" {
        # "Template Separator\n(You can make a copy of, or modify, this frame)"
        n129 = Unbundle By Name(w325) -> ("Source Voltage"=w334:dbl, "Final Temp"=w332:i32, "Init Temp"=w329:i32, "Temp Step"=w328:i32, "Data File"=w330:path, "Trimming"=w327:i32)
        n130 = Subtract(x=w332, y=w329) -> (x-y=w335:i32)
        n131 = Divide(x=w335, y=w328) -> (x/y=w336:dbl)
        n132 = Increment(x=w336) -> (x+1=w331:dbl)
        n133 = for {
          N: w331 -> [_]
          tunnel: w334 -> [w340]
          tunnel: [w351] -> w333 mode=indexing
          tunnel: w330 -> [w350]
          tunnel: w329 -> [w349]
          tunnel: w328 -> [w348]
          tunnel: w327 -> [w347]
          i -> [w354]
          n134 = Strip Path(path=w350) -> (stripped path=w359:path, name=w358:string)
          n135 = Multiply(x=w348, y=w354) -> (x*y=w355:i32)
          n136 = Add(x=w349, y=w355) -> (x+y=w360:i32)
          n137 = String Subset(string=w358, length (rest)=18) -> (substring=w356:string)  [unwired: 1 in]
          n138 = Format Into String(w360) -> (resulting string=w362:string)  [unwired: 3 in, 1 out]
          n139 = Concatenate Strings(w356, w362, "K.dat" ("string")) -> (w361:string)
          n140 = call-poly <userlib>:"Build Path__ogtk.vi"("name or relative path"=w361, "base path"=w359) -> ("appended path"=w363:path)
          n141 = call <userlib>:"Data Read.vi"("path"=w363) -> ("Data (Dictionary)"=w345:T6[])  [unwired: 7 in, 3 out]
          n142 = call "Read Dictionary.vi"("Numeric"=0, "Dictionary In"=w345) -> ("data"=w344:dbl[])
          n143 = call "Read Dictionary.vi"("Numeric"=10, "Dictionary In"=w345) -> ("data"=w343:dbl[])
          n144 = Array Subset(array=w344, index=w347) -> (w346:dbl[])  [unwired: 1 in]
          n145 = Array Subset(array=w343, index=w347) -> (w339:dbl[])  [unwired: 1 in]
          n146 = Absolute Value(x=w339) -> (abs(x)=w338:dbl[])
          n147 = Divide(x=w338, y=w340) -> (x/y=w353:dbl[])
          n148 = Bundle(w346, w353) -> (w351:cluster{dbl[], dbl[]})  [unwired: 1 in]
        }
        n149 = call <vilib>:"Add State(s) to Queue__jki_lib_state_machine.vi"("State(s) in (\"\")"=w323) -> ("States Out"=w324:string)  [unwired: 14 in]
        n150 = Bundle By Name(cluster=w325, "G2T BG"=w333) -> (w326:T4)
      }
      frame "Analysis: Plot G vs t" {
        n151 = Unbundle By Name(w370) -> ("G2T 1D"=→"G2T vs t":cluster{dbl[], dbl[]}[], "G4T 1D"=→"G4T vs t":cluster{dbl[], dbl[]}[], "G2T 2D"=→"G2T vs t 2D":cluster{dbl[], dbl[]}[], "G4T 2D"=→"G4T vs t  2D":cluster{dbl[], dbl[]}[], "G2T BG"=→"G2T BG vs t":cluster{dbl[], dbl[]}[], "Temp"=→"Temp vs t":cluster{dbl[], dbl[]}[])
        n152 = call <vilib>:"Add State(s) to Queue__jki_lib_state_machine.vi"("State(s) in (\"\")"=w373) -> ("States Out"=w372:string)  [unwired: 14 in]
      }
      frame "Analysis: Arrhenius Plot" {
        n153 = Unbundle By Name(w414) -> ("G2T 1D"=w377:cluster{dbl[], dbl[]}[], "G4T 1D"=w376:cluster{dbl[], dbl[]}[], "G2T 2D"=w383:cluster{dbl[], dbl[]}[], "G4T 2D"=w385:cluster{dbl[], dbl[]}[], "Final Temp"=w411:i32, "Init Temp"=w409:i32, "Temp Step"=w408:i32)  [unwired: 1 out]
        n154 = Subtract(x=w411, y=w409) -> (x-y=w412:i32)
        n155 = Divide(x=w412, y=w408) -> (x/y=w413:dbl)
        n156 = Increment(x=w413) -> (x+1=w410:dbl)
        n157 = for {
          N: w410 -> [_]
          tunnel: w409 -> [w420]
          tunnel: w408 -> [w421]
          tunnel: [w418] -> w394 mode=indexing
          i -> [w422]
          n158 = Multiply(x=w421, y=w422) -> (x*y=w423:i32)
          n159 = Add(x=w420, y=w423) -> (x+y=w419:i32)
          n160 = Reciprocal(x=w419) -> (1/x=w418:dbl)
        }
        n161 = call-poly <userlib>:"Linear Fit.vi"("XY-data"=w377) -> ("slopes"=w374:dbl[])  [unwired: 4 in, 6 out]
        n162 = call-poly <userlib>:"Linear Fit.vi"("XY-data"=w376) -> ("slopes"=w375:dbl[])  [unwired: 4 in, 6 out]
        n163 = call-poly <userlib>:"Linear Fit.vi"("XY-data"=w383) -> ("slopes"=w382:dbl[])  [unwired: 4 in, 6 out]
        n164 = call-poly <userlib>:"Linear Fit.vi"("XY-data"=w385) -> ("slopes"=w384:dbl[])  [unwired: 4 in, 6 out]
        n165 = Absolute Value(x=w374) -> (abs(x)=w404:dbl[])
        n166 = Absolute Value(x=w375) -> (abs(x)=w405:dbl[])
        n167 = Absolute Value(x=w382) -> (abs(x)=w406:dbl[])
        n168 = Absolute Value(x=w384) -> (abs(x)=w407:dbl[])
        n169 = Natural Logarithm(1:w404) -> (0:w398:dbl[])
        n170 = Natural Logarithm(1:w405) -> (0:w397:dbl[])
        n171 = Natural Logarithm(1:w406) -> (0:w396:dbl[])
        n172 = Natural Logarithm(1:w407) -> (0:w395:dbl[])
        n173 = Array Subset(array=w398, length="Temps to keep (Arrhenius fit)") -> (w392:dbl[])  [unwired: 1 in]
        n174 = Array Subset(array=w397, length="Temps to keep (Arrhenius fit)") -> (w391:dbl[])  [unwired: 1 in]
        n175 = Array Subset(array=w396, length="Temps to keep (Arrhenius fit)") -> (w390:dbl[])  [unwired: 1 in]
        n176 = Array Subset(array=w395, length="Temps to keep (Arrhenius fit)") -> (w389:dbl[])  [unwired: 1 in]
        n177 = Array Subset(array=w394, length="Temps to keep (Arrhenius fit)") -> (w388:dbl[])  [unwired: 1 in]
        n178 = Bundle(w388, w392) -> (w401:cluster{dbl[], dbl[]})  [unwired: 1 in]
        n179 = Bundle(w388, w391) -> (w403:cluster{dbl[], dbl[]})  [unwired: 1 in]
        n180 = Bundle(w388, w390) -> (w402:cluster{dbl[], dbl[]})  [unwired: 1 in]
        n181 = Bundle(w388, w389) -> (w400:cluster{dbl[], dbl[]})  [unwired: 1 in]
        n182 = Build Array(w401, w403, w402, w400) -> (w381:cluster{dbl[], dbl[]}[])
        n183 = call-poly <userlib>:"Linear Fit.vi"("XY-data"=w381) -> ("Best Fits"=w380:cluster{"X-array":dbl[], "Y-array":dbl[]}[], "XY-data out"=w379:cluster{"X-array":dbl[], "Y-array":dbl[]}[], "slopes"=w378:dbl[])  [unwired: 4 in, 4 out]
        n184 = Multiply(x=w378, y=8.617333e-05) -> (x*y=→"E_a":dbl[])
        n185 = Interleave 1D Arrays(w379, w380) -> (→"Arrhenius":cluster{"X-array":dbl[], "Y-array":dbl[]}[])
        n186 = call <vilib>:"Add State(s) to Queue__jki_lib_state_machine.vi"("State(s) in (\"\")"=w417) -> ("States Out"=w416:string)  [unwired: 14 in]
      }
      frame "Analysis: Lifespan" {
        w432 = 3600
        # "Template Separator\n(You can make a copy of, or modify, this frame)"
        n187 = Unbundle By Name(w454) -> ("G2T 1D"=w471:cluster{dbl[], dbl[]}[], "G4T 1D"=w470:cluster{dbl[], dbl[]}[], "G2T 2D"=w469:cluster{dbl[], dbl[]}[], "G4T 2D"=w468:cluster{dbl[], dbl[]}[], "Final Temp"=w465:i32, "Init Temp"=w453:i32, "Temp Step"=w452:i32)  [unwired: 1 out]
        n188 = Subtract(x=w465, y=w453) -> (x-y=w466:i32)
        n189 = Divide(x=w466, y=w452) -> (x/y=w467:dbl)
        n190 = Increment(x=w467) -> (x+1=w451:dbl)
        n191 = for {
          N: w451 -> [_]
          tunnel: w453 -> [w489]
          tunnel: w452 -> [w488]
          tunnel: [w487] -> w450 mode=indexing
          i -> [w490]
          n192 = Multiply(x=w488, y=w490) -> (x*y=w491:i32)
          n193 = Add(x=w489, y=w491) -> (x+y=w487:i32)
        }
        n194 = call <userlib>:"Linear Fit (multiple).vi"("XY-data"=w471) -> ("XY-data out"=w445:cluster{"X-array":dbl[], "Y-array":dbl[]}[], "slopes"=w448:dbl[])  [unwired: 4 in, 5 out]
        n195 = call <userlib>:"Linear Fit (multiple).vi"("XY-data"=w470) -> ("XY-data out"=w444:cluster{"X-array":dbl[], "Y-array":dbl[]}[], "slopes"=w447:dbl[])  [unwired: 4 in, 5 out]
        n196 = call <userlib>:"Linear Fit (multiple).vi"("XY-data"=w469) -> ("XY-data out"=w443:cluster{"X-array":dbl[], "Y-array":dbl[]}[], "slopes"=w446:dbl[])  [unwired: 4 in, 5 out]
        n197 = call <userlib>:"Linear Fit (multiple).vi"("XY-data"=w468) -> ("XY-data out"=w442:cluster{"X-array":dbl[], "Y-array":dbl[]}[], "slopes"=w449:dbl[])  [unwired: 4 in, 5 out]
        n198 = for {
          tunnel: w445 -> [w483] mode=indexing
          tunnel: w444 -> [w484] mode=indexing
          tunnel: w443 -> [w485] mode=indexing
          tunnel: w442 -> [w486] mode=indexing
          tunnel: [w478] -> w441 mode=indexing
          tunnel: [w477] -> w440 mode=indexing
          tunnel: [w476] -> w439 mode=indexing
          tunnel: [w475] -> w438 mode=indexing
          n199 = Unbundle(w483) -> ("Y-array"=w479:dbl[])  [unwired: 1 out]
          n200 = Unbundle(w484) -> ("Y-array"=w480:dbl[])  [unwired: 1 out]
          n201 = Unbundle(w485) -> ("Y-array"=w481:dbl[])  [unwired: 1 out]
          n202 = Unbundle(w486) -> ("Y-array"=w482:dbl[])  [unwired: 1 out]
          n203 = call-poly <vilib>:"Mean.vi"("X"=w482) -> ("mean"=w475:dbl)  [unwired: 1 out]
          n204 = call-poly <vilib>:"Mean.vi"("X"=w481) -> ("mean"=w476:dbl)  [unwired: 1 out]
          n205 = call-poly <vilib>:"Mean.vi"("X"=w480) -> ("mean"=w477:dbl)  [unwired: 1 out]
          n206 = call-poly <vilib>:"Mean.vi"("X"=w479) -> ("mean"=w478:dbl)  [unwired: 1 out]
        }
        n207 = Divide(x=w441, y=w448) -> (x/y=w436:dbl[])
        n208 = Divide(x=w440, y=w447) -> (x/y=w435:dbl[])
        n209 = Divide(x=w439, y=w446) -> (x/y=w434:dbl[])
        n210 = Divide(x=w438, y=w449) -> (x/y=w433:dbl[])
        n211 = Divide(x=w436, y=w432) -> (x/y=w428:dbl[])
        n212 = Divide(x=w435, y=w432) -> (x/y=w429:dbl[])
        n213 = Divide(x=w434, y=w432) -> (x/y=w430:dbl[])
        n214 = Divide(x=w433, y=w432) -> (x/y=w431:dbl[])
        n215 = Array Subset(array=w428, length="Temps to keep (Lifespan)") -> (w459:dbl[])  [unwired: 1 in]
        n216 = Array Subset(array=w429, length="Temps to keep (Lifespan)") -> (w458:dbl[])  [unwired: 1 in]
        n217 = Array Subset(array=w430, length="Temps to keep (Lifespan)") -> (w457:dbl[])  [unwired: 1 in]
        n218 = Array Subset(array=w431, length="Temps to keep (Lifespan)") -> (w456:dbl[])  [unwired: 1 in]
        n219 = Array Subset(array=w450, length="Temps to keep (Lifespan)") -> (w455:i32[])  [unwired: 1 in]
        n220 = Absolute Value(x=w459) -> (abs(x)=w424:dbl[])
        n221 = Absolute Value(x=w458) -> (abs(x)=w425:dbl[])
        n222 = Absolute Value(x=w457) -> (abs(x)=w426:dbl[])
        n223 = Absolute Value(x=w456) -> (abs(x)=w427:dbl[])
        n224 = Bundle(w455, w424) -> (w462:cluster{i32[], dbl[]})  [unwired: 1 in]
        n225 = Bundle(w455, w425) -> (w464:cluster{i32[], dbl[]})  [unwired: 1 in]
        n226 = Bundle(w455, w426) -> (w463:cluster{i32[], dbl[]})  [unwired: 1 in]
        n227 = Bundle(w455, w427) -> (w461:cluster{i32[], dbl[]})  [unwired: 1 in]
        n228 = Build Array(w462, w464, w463, w461) -> (→"Lifespan vs Temp (hrs)":cluster{i32[], dbl[]}[])
        n229 = call <vilib>:"Add State(s) to Queue__jki_lib_state_machine.vi"("State(s) in (\"\")"=w474) -> ("States Out"=w473:string)  [unwired: 14 in]
      }
    }
  }
  "error out" <- w1
